vi "Check Error Status.vi"(8 "error in (no error)":errorcluster, 10 "Current Code":i32, 11 "Previous Code":i32) -> (0 "Error out":errorcluster, 3 "Send Alarm":bool)   [LabVIEW 2020]
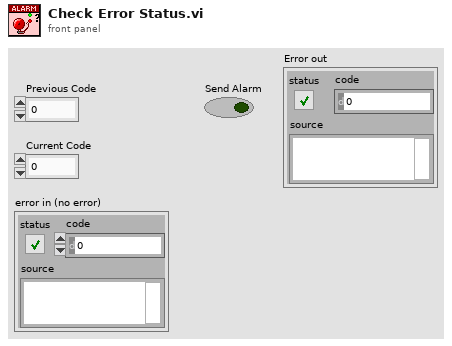
[diagram p1: front panel]
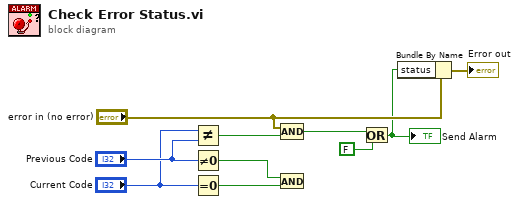
[diagram p0: block diagram]
diagram:
  n1 = Not Equal?(x="Current Code", y="Previous Code") -> (x != y?=w1:bool)
  n2 = Not Equal To 0?(x="Previous Code") -> (x != 0?=w10:bool)
  n3 = Equal To 0?(x="Current Code") -> (x = 0?=w9:bool)
  n4 = And(x=w10, y=w9) -> ()  [unwired: 1 out]
  n5 = Compound Arithmetic op=AND("error in (no error)", w1) -> (w6:bool)
  n6 = Or(x=w6, y=FALSE) -> (x .or. y?=w4:bool)
  "Send Alarm" <- w4
  n7 = Bundle By Name(cluster="error in (no error)", "status"=w4) -> (→"Error out":errorcluster)
